vi "Create Log or Log Directory.vi"(0 "Base Directory":path, 1 "Run":i32=1, 2 "Subrun":i32=1, 3 "Append if exists?":bool, 4 "Log Type":T1, 5 "error in":errorcluster) -> (14 "Path":path, 19 "error out":errorcluster)   [LabVIEW 2018]
uses:
  logs.ctl
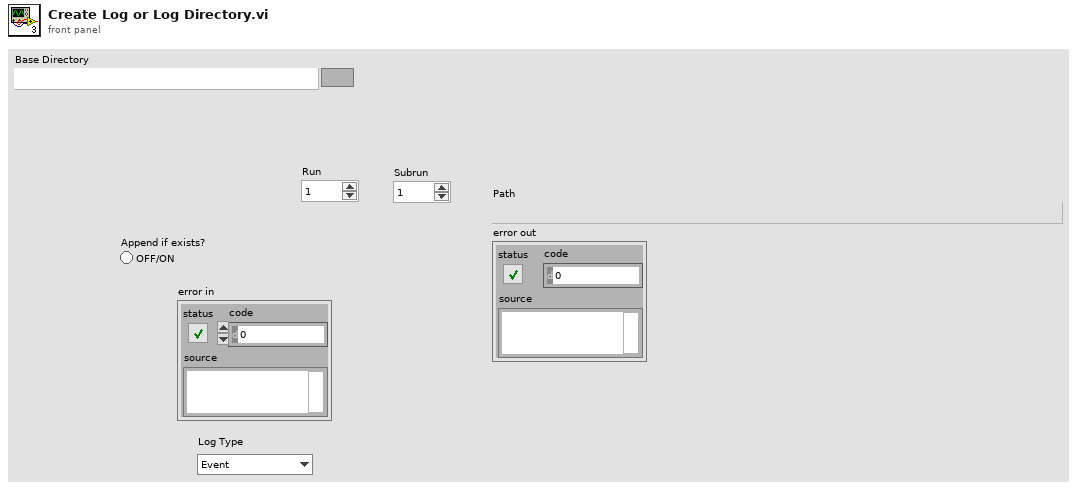
[diagram p1: front panel]
types:
  T1 = typedef "logs.ctl" = enum16{"Event", "ZMQ", "Channel", "Program"}
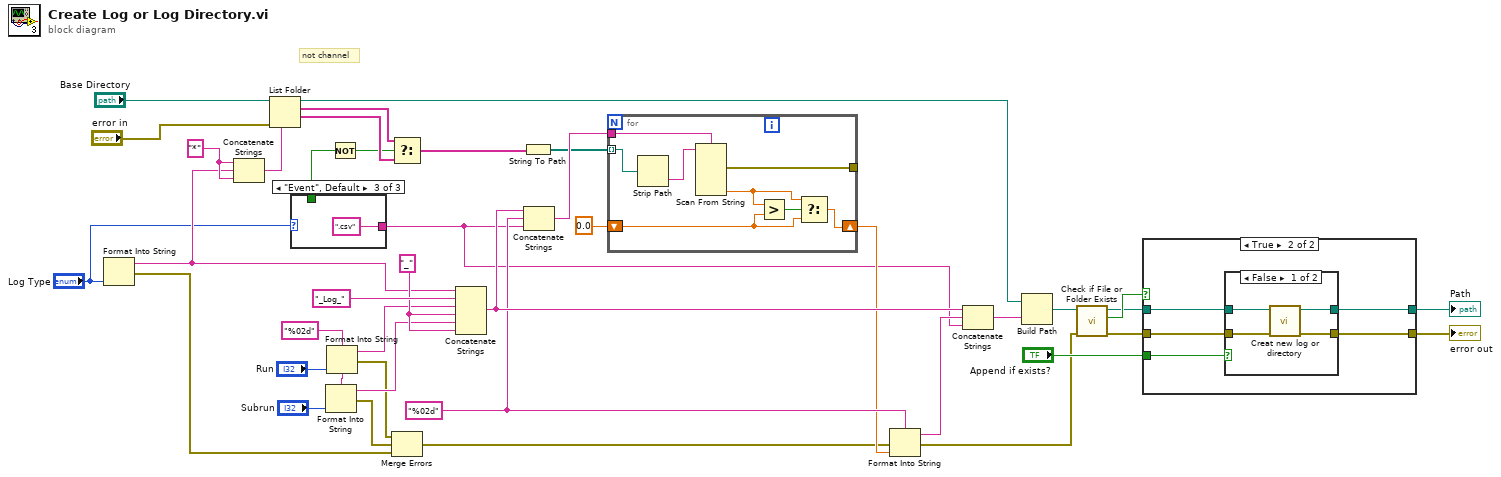
[diagram p0: block diagram]
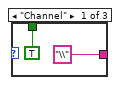
[diagram p2: hidden frame]
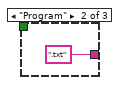
[diagram p3: hidden frame]
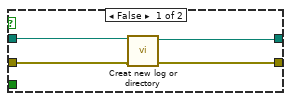
[diagram p4: hidden frame]
diagram:
  w8 = "%02d" ("string")
  w28 = "*" ("string")
  w19 = "%02d" ("format string")
  w39 = "_" ("string")
  # "not channel"
  n1 = Format Into String("Log Type") -> (resulting string=w5:string, error out=w12:errorcluster)  [unwired: 3 in]
  n2 = Concatenate Strings(w28, w5, w28) -> (w27:string)
  n3 = List Folder(path="Base Directory", pattern=w27, error in="error in") -> (path out=w26:path, filenames=w25:string[], folder names=w24:string[])  [unwired: 1 in, 1 out]
  n4 = case shown="\"Event\", Default" "Log Type" {
    tunnel: ["\\" ("string") ".txt" ("string") ".csv" ("string")] -> w3
    tunnel: [TRUE ("s") _ _] -> w2
    frame "Channel" {
    }
    frame "Program" {
    }
    frame "Event", Default {
    }
  }
  n5 = Format Into String(format string=w8, "Subrun") -> (resulting string=w13:string, error out=w9:errorcluster)  [unwired: 2 in]
  n6 = Format Into String(format string=w8, "Run") -> (resulting string=w14:string, error out=w10:errorcluster)  [unwired: 2 in]
  n7 = Not(x=w2) -> (.not. x?=w1:bool)
  n8 = Select(t=w25, s=w1, f=w24) -> (s? t:f=w7:string[])
  n9 = Merge Errors(w10, w9, w12) -> (w11:errorcluster)
  n10 = Concatenate Strings(w5, "_Log_" ("string"), w14, w39, w13, w39) -> (w20:string)
  n11 = String To Path(string=w7) -> (path=w6:path[])
  n12 = Concatenate Strings(w20, w19, w3) -> (w18:string)
  n13 = for {
    tunnel: w6 -> [w46] mode=indexing
    shift-right: [w47] -> w17
    shift-left: 0.0 ("Subrun") -> [w49]
    tunnel: [w52] -> _
    tunnel: w18 -> [w51]
    n14 = Strip Path(path=w46) -> (name=w45:string)  [unwired: 1 out]
    n15 = Scan From String(format string=w51, input string=w45) -> (error out=w52:errorcluster, output 3=w48:dbl)  [unwired: 7 in, 2 out]
    n16 = Greater?(x=w48, y=w49) -> (0:w50:bool)
    n17 = Select(t=w48, s=w50, f=w49) -> (s? t:f=w47:dbl)
  }
  n18 = Format Into String(format string=w19, error in=w11, w17) -> (resulting string=w21:string, error out=w29:errorcluster)  [unwired: 1 in]
  n19 = Concatenate Strings(w20, w21, w3) -> (w22:string)
  n20 = Build Path(base path=w26, name or relative path=w22) -> (appended path=w34:path)
  n21 = call <vilib>:"Check if File or Folder Exists.vi"("error in (no error)"=w29, "path"=w34) -> ("error out"=w36:errorcluster, "file or folder exists?"=w38:bool, "dup path"=w37:path)  [unwired: 7 in]
  n22 = case shown="True" w38 {
    tunnel: [w54 w58] -> w32
    tunnel: [w55 w59] -> w33
    tunnel: w37 -> [w56 w60]
    tunnel: w36 -> [w53 w57]
    tunnel: "Append if exists?" -> [_ w61]
    frame False {
      n23 = call "Creat new log or directory.vi"("error in"=w53, "Log"=w56) -> ("error out"=w54:errorcluster, "New Log"=w55:path)  [unwired: 8 in]
    }
    frame True {
      n24 = case shown="False" w61 {
        tunnel: w60 -> [w64 w67]
        tunnel: [w63 w67] -> w59
        tunnel: [w62 w66] -> w58
        tunnel: w57 -> [w65 w66]
        frame False {
          n25 = call "Creat new log or directory.vi"("error in"=w65, "Log"=w64) -> ("error out"=w62:errorcluster, "New Log"=w63:path)  [unwired: 8 in]
        }
        frame True {
        }
      }
    }
  }
  "Path" <- w33
  "error out" <- w32
